vi "Configuration Utility.vi"() -> ()   [LabVIEW 2013, in "configuration library.lvlib"]
doc: "This is the main VI for the configuration editor."
uses:
  configuration library.lvlib
  Controls/StateCluster.ctl
  <vilib>/NI/Tag Bus Data Framework/Configuration Editor/Classes/SystemConfigRepo/SystemConfigRepo.lvclass
  <vilib>/NI/Configuration Framework/Node/NodeRef.ctl
  <vilib>/NI/Configuration Framework/Node/NISE_CEF_Node.lvclass
  subVI/SplashScreen/splash screen.ctl
  subVI/SplashScreen/notifier data.ctl
  <vilib>/NI/Configuration Framework/Node/StandardEvents.ctl
  <vilib>/NI/Configuration Framework/Node/UserEventRef.ctl
  <vilib>/NI/Configuration Framework/Controls/EventCluster.ctl
  <vilib>/NI/Configuration Framework/Node/NodeChangeEvent.ctl
  <vilib>/NI/Configuration Framework/Node/CacheState.ctl
  <vilib>/NI/Configuration Framework/Node/RefreshUIEvent.ctl
  <vilib>/NI/Configuration Framework/Node/StopEvent.ctl
  <vilib>/NI/Configuration Framework/glyph manager/glyph manager.ctl
  <vilib>/picture/picture.llb/imagedata.ctl
  Controls/add message.ctl
  Controls/MoveMessage.ctl
  <vilib>/NI/Tag Bus Data Framework/Configuration Editor/Classes/Systems/Systems.lvclass
  <vilib>/NI/Configuration Framework/Repository/NISE_CEF_Repository.lvclass
  <vilib>/NI/AMC/Create Single Message.vi
  <vilib>/NI/AMC/Update Message Routing Info.vi
  <vilib>/NI/AMC/Read Termination Message.vi
  <vilib>/NI/Tag Bus Data Framework/Configuration Editor/subVIs/Glyphs Status.ctl
  <vilib>/NI/Tag Bus Data Framework/Configuration Editor/subVIs/Add status to name.vi
  <vilib>/NI/AMC/Send Message.vi
  <vilib>/NI/AMC/Globals.vi
  <vilib>/NI/Tag Bus Data Framework/Configuration Editor/Classes/Module editor node/module editor node.lvclass
  <vilib>/NI/Tag Bus Data Framework/Configuration Editor/Classes/EngineTags/EngineTags.lvclass
  <vilib>/NI/Module Timing Source/timing source/TBM timing source.lvclass
  <vilib>/NI/Tag Bus Data Framework/Configuration Editor/Classes/TBM Configuration Node/TBM Configuration Node.lvclass
  <vilib>/NI/Tag Bus Module Framework/root configuration/TBM configuration.lvclass
  <vilib>/NI/Tag Bus Data Framework/Framework Configuration Classes/target configuration/PL_Target Configuration.lvclass
  <vilib>/NI/Tag Bus Data Framework/Configuration Editor/Classes/Targets/Targets.lvclass
  <vilib>/NI/Tag Bus Data Framework/Configuration Editor/Classes/Engine Parent/Engine Parent Editor Node.lvclass
  <vilib>/NI/Tag Bus Data Framework/Framework Configuration Classes/system configuration/PL_System Configuration.lvclass
  <vilib>/NI/Module Execution Interface/Engine Configuration/engine configuration.lvclass
  <vilib>/NI/Tag Bus Module Framework/channel/TBM channel.lvclass
  <vilib>/NI/Tag Bus Module Framework/module configuration/TBM module configuration.lvclass
  <vilib>/NI/AMC/AMC.lvlib
  <vilib>/NI/Configuration Framework/NISE_CEF_TreeControl.lvlib
  subVI/SplashScreen/splash screen.lvlib
  <vilib>/NI/Tag Bus Data Framework/Framework Configuration Classes/class cache/PL_class cache.lvlib
  <vilib>/NI/Tag Bus Data Framework/Configuration Editor/PL Framework Configuration Tool.lvlib
  <vilib>/NI/Configuration Framework/hierarchy repo/NISE_CEF_HierarchyRepo.lvclass
  <vilib>/NI/Configuration Framework/tree serializer/NISE_CEF_TreeSerializer.lvlib
  <vilib>/NI/Configuration Framework/glyph manager/glyph manager.lvlib
panel:
  in  "Exit":bool
  in  "View":string(tree)
  # "Tag Bus Configuration Editor"
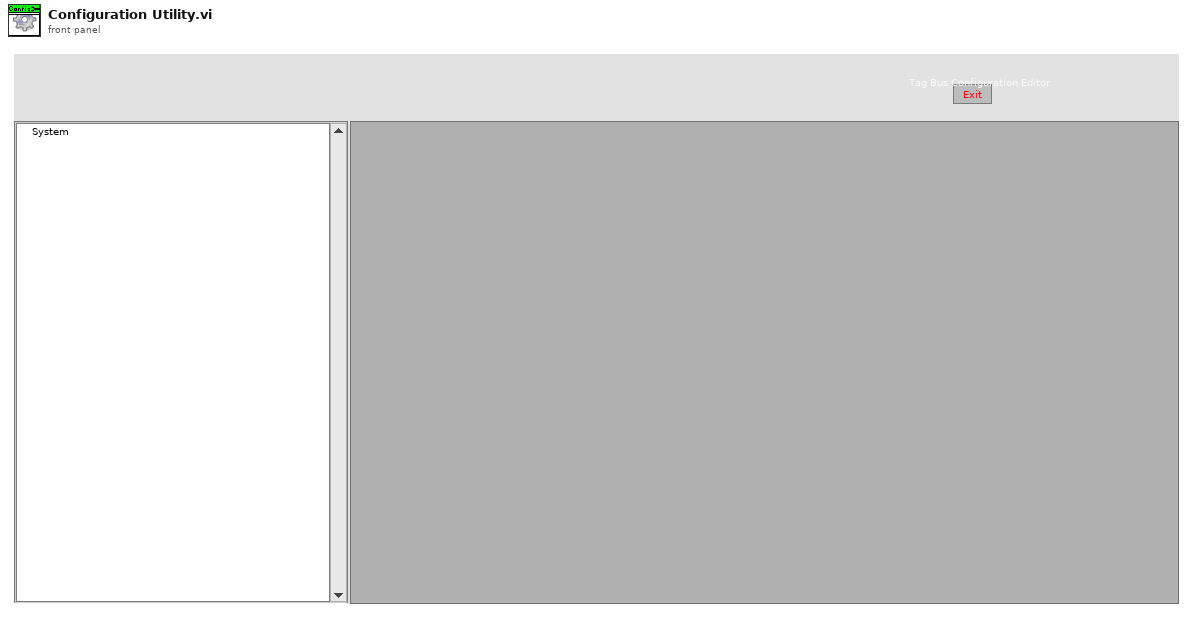
[diagram p1: front panel]
types:
  T1 = enum32{"Invalid", "Standard", "Closed", "Hidden", "Minimized", "Maximized"}
  T2 = typedef "configuration library.lvlib/StateCluster.ctl" = cluster{"repository":refnum<class "SystemConfigRepo.lvclass">, "root":T3, "unsaved changes":bool, "current path":path, "SplashScreen":T4, "classes cache":path, "standard events":T5, "glyph manager":T11}
  T3 = typedef "NISE_CEF_Node.lvclass/NodeRef.ctl" = refnum<data-value>
  T4 = typedef "configuration library.lvlib/splash screen.lvlib/splash screen.ctl" = cluster{"reference":refnum<vi>, "update notifier":refnum<notifier>, "Initialized":bool}
  T5 = typedef "NISE_CEF_Node.lvclass/StandardEvents.ctl" = cluster{"user event":T6, "node change":T7, "cache state":T8, "refresh UI":T9, "stop event":T10}
  T6 = typedef "NISE_CEF_Node.lvclass/UserEventRef.ctl" = refnum<user-event>
  T7 = typedef "NISE_CEF_Node.lvclass/NodeChangeEvent.ctl" = refnum<user-event>
  T8 = typedef "NISE_CEF_Node.lvclass/CacheState.ctl" = refnum<user-event>
  T9 = typedef "NISE_CEF_Node.lvclass/RefreshUIEvent.ctl" = refnum<user-event>
  T10 = typedef "NISE_CEF_Node.lvclass/StopEvent.ctl" = refnum<user-event>
  T11 = typedef "glyph manager.lvlib/glyph manager.ctl" = cluster{"search paths":path[], "glyph map":variant, "base glyphs":T12[], "desired overlays":string[]}
  T12 = typedef "imagedata.ctl" = cluster{"image type":i32, "image depth":i32, "image":u8[], "mask":u8[], "colors":u32[], "Rectangle":cluster{"left":i16, "top":i16, "right":i16, "bottom":i16}}
  T13 = typedef "AMC.lvlib/Message Queue.ctl" = refnum<queue>
  T14 = typedef "configuration library.lvlib/splash screen.lvlib/notifier data.ctl" = cluster{"Text":string, "percent":dbl}
  T15 = cluster{"node id":string, "RightClickPath":string}
  T16 = typedef "configuration library.lvlib/add message.ctl" = cluster{"node type":string, "to add to":string}
  T17 = typedef "configuration library.lvlib/MoveMessage.ctl" = cluster{"node ref":T3, "new parent":T3}
  T18 = typedef "configuration library.lvlib/FilePaths.ctl" = cluster{"glyphs":path[], "classes":path, "classes cache":path}
  T19 = typedef "PL_class cache.lvlib/cache definition.ctl" = cluster{"configuration":T20, "class cache data":T21}
  T20 = typedef "PL_class cache.lvlib/cache search configuration.ctl" = cluster{"Search Paths":path[], "Folders to Exclude":string[], "full class list":path[]}
  T21 = typedef "PL_class cache.lvlib/cached class information.ctl" = cluster{"targets":T22[], "engines":T23[], "modules":T23[], "ignored class list":path[]}
  T22 = typedef "PL_class cache.lvlib/target class metadata.ctl" = cluster{"file name":string, "fully qualified name":string, "menu display name":string, "configuration class name":string}
  T23 = typedef "PL_class cache.lvlib/class metadata.ctl" = cluster{"file name":string, "fully qualified name":string, "menu display name":string, "configuration class":string, "instances allowed":i32, "supported targets":T24[]}
  T24 = typedef "TBM configuration.lvclass/Target Types.ctl" = enum16{"Windows", "Mac", "Linux", "Linux RT ARM", "VxWorks", "Pharlap", "Other", "Linux RT x64"}
  T25 = typedef "NISE_CEF_Node.lvclass/Summary.ctl" = cluster{"ID":string, "parent ID":string, "node type":string, "text":string, "additional text":string, "glyph":string, "depth":i32, "glyph overlay":string}
  T26 = typedef "LVPoint32TypeDef.ctl" = cluster{"Horizontal":i32, "Vertical":i32}
  T27 = cluster{"data name":string, "drag data":variant}[]
  T28 = typedef "NISE_CEF_Node.lvclass/NodeMenuOptions.ctl" = cluster{"removable":bool, "movable":bool, "duplicate":bool}
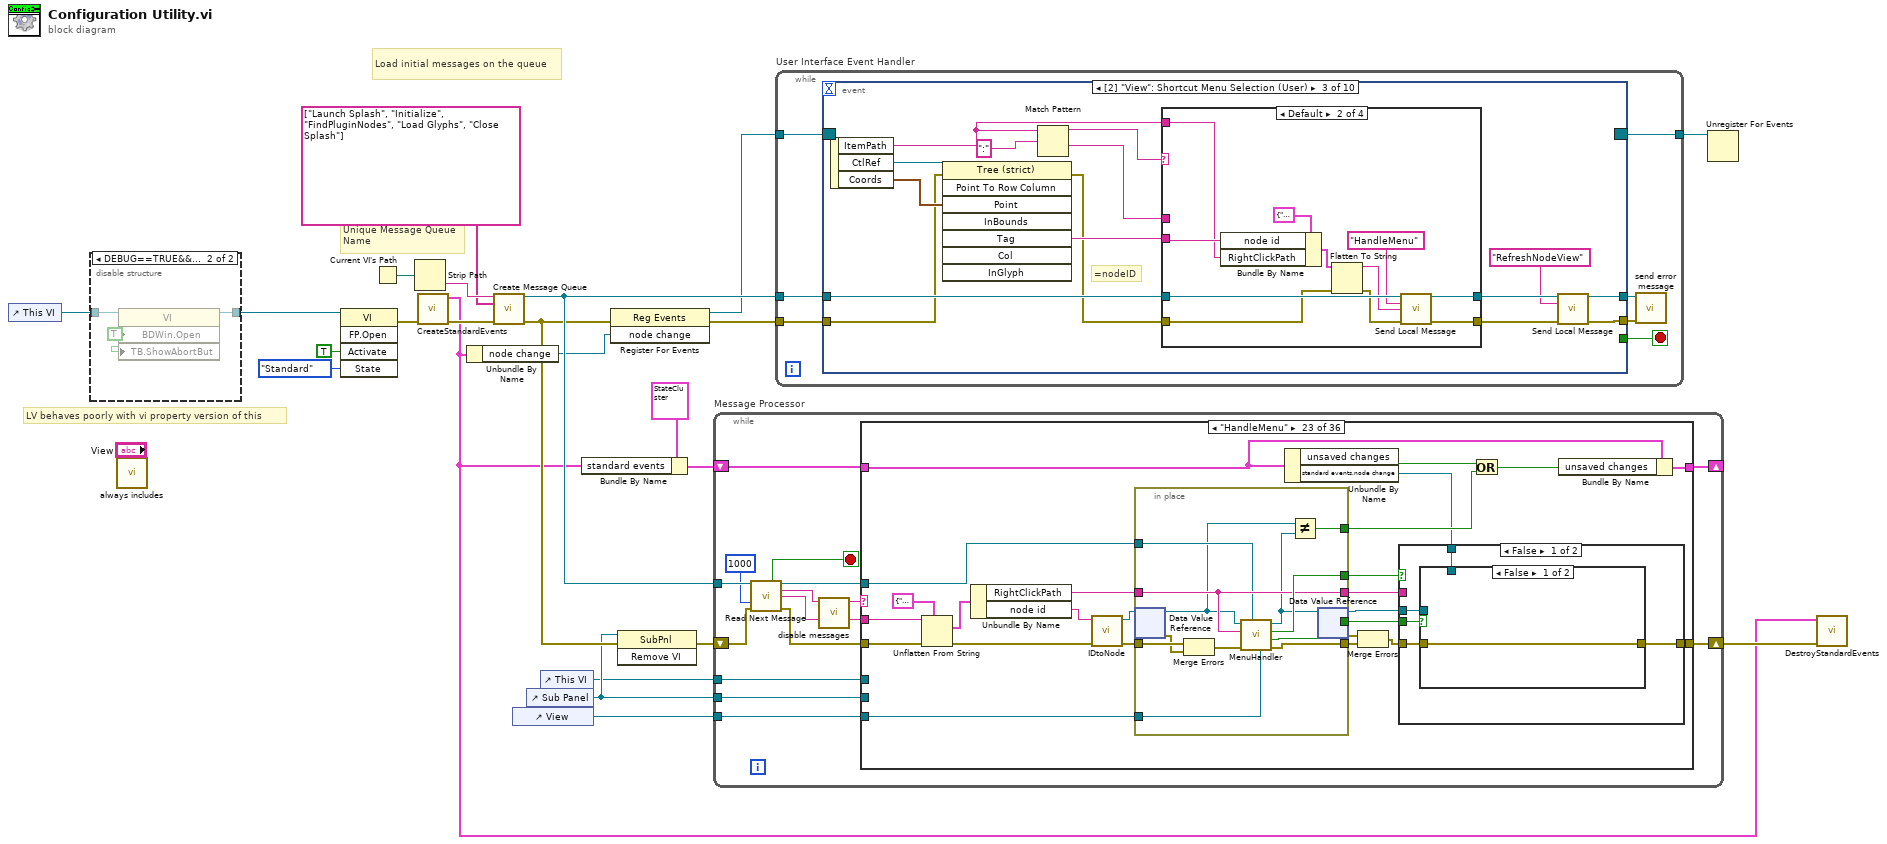
[diagram p0: block diagram]
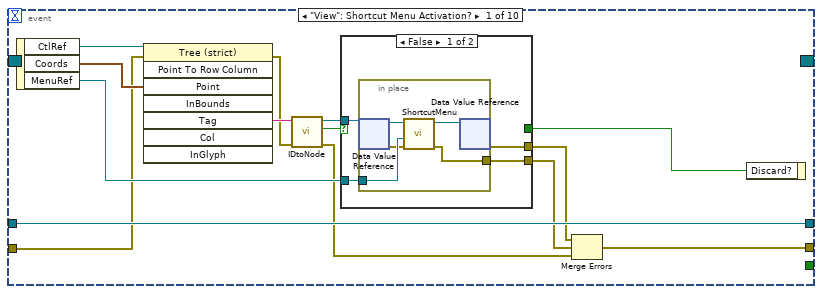
[diagram p3: hidden frame]
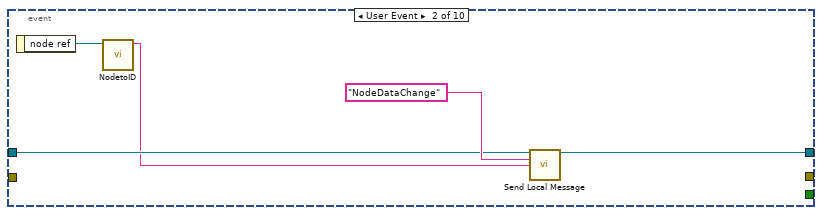
[diagram p5: hidden frame]
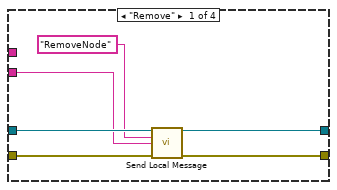
[diagram p6: hidden frame]
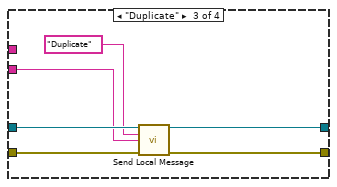
[diagram p7: hidden frame]
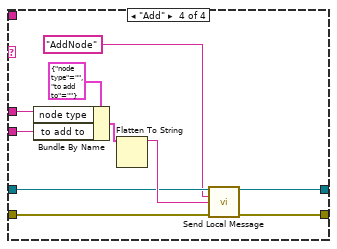
[diagram p8: hidden frame]
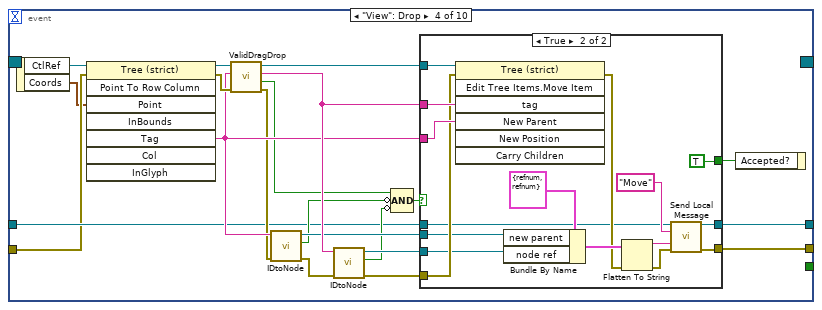
[diagram p9: hidden frame]
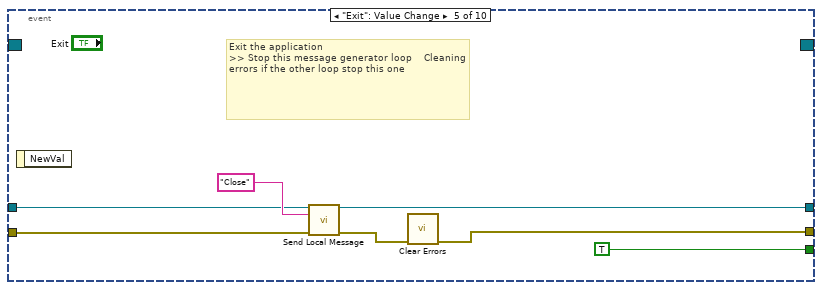
[diagram p11: hidden frame]
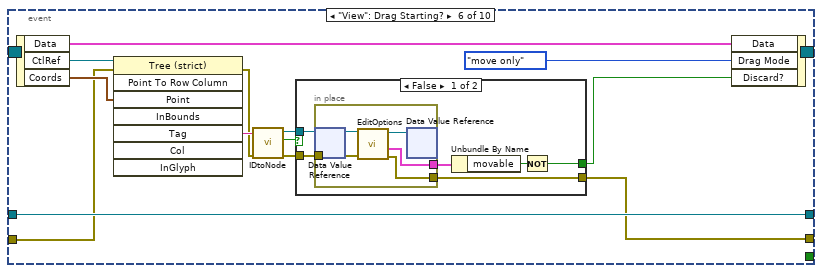
[diagram p12: hidden frame]
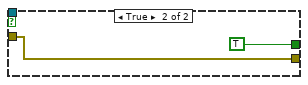
[diagram p13: hidden frame]
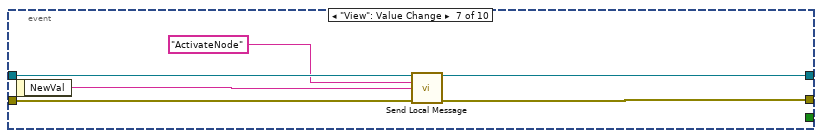
[diagram p14: hidden frame]
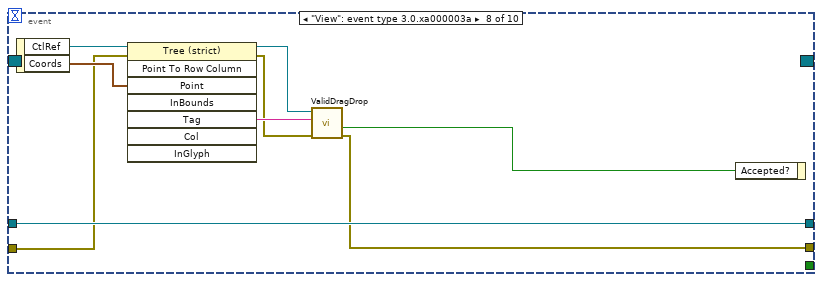
[diagram p15: hidden frame]
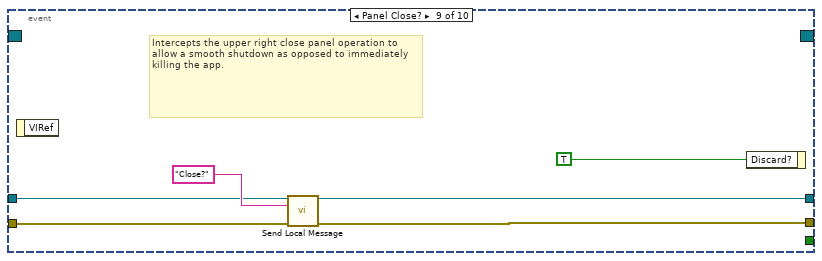
[diagram p16: hidden frame]
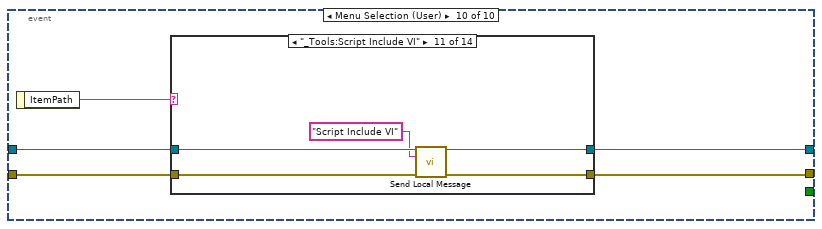
[diagram p17: hidden frame]
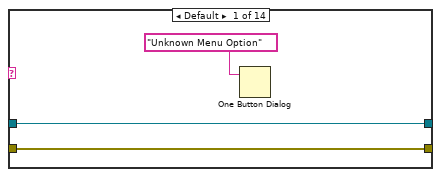
[diagram p18: hidden frame]
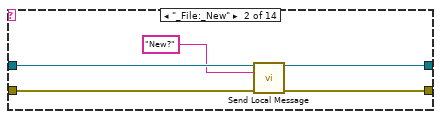
[diagram p19: hidden frame]
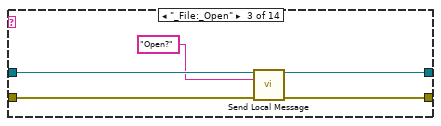
[diagram p20: hidden frame]
diagram:
  # "LV behaves poorly with vi property version of this"
  # "Unique Message Queue Name"
  # "Load initial messages on the queue"
  n1 = control-ref of="This VI"() -> (w14:refnum<vi>)
  n2 = disable-structure shown="DEBUG==TRUE&&RUN_TIME_ENGINE==False" {
    disable-tunnel: [w24 w27] -> w15
    disable-tunnel: w14 -> [w24 w26]
    frame condition #0 (active) {
    }
    frame condition #1 {
      w25 = TRUE ("Block Diagram Window:Open")
      n3 = property class="VI"(reference=w26, "BDWin.Open"=w25, "TB.ShowAbortBut"=w25) -> (reference out=w27:refnum<vi>)  [unwired: 1 in, 1 out]
    }
  }
  n4 = call "always includes.vi"() -> ()  [unwired: 12 in]
  n5 = invoke class="VI" method="FP.Open"(reference=w15, "Activate"=TRUE ("Activate?"), "State"=T1."Standard") -> (error out=w9:errorcluster)  [unwired: 2 in, 4 out]
  n6 = Current VI's Path() -> (path=w22:path)
  n7 = Strip Path(path=w22) -> (name=w23:string)  [unwired: 1 out]
  n8 = call <vilib>:"CreateStandardEvents.vi"("error in"=w9) -> ("error out"=w8:errorcluster, "standard events"=w1:T5)  [unwired: 9 in]
  n9 = Unbundle By Name(w1) -> ("node change"=w6:T7)
  n10 = call <vilib>:"Create Message Queue.vi"("message queue name"=w23, "initial message names"=string[] ["Launch Splash", "Initialize", "FindPluginNodes", "Load Glyphs", "Close Splash"], "error in"=w8) -> ("message queue out"=w20:T13, "error out"=w18:errorcluster)  [unwired: 11 in]
  n11 = control-ref of="View"() -> (w13:refnum<vi>)
  n12 = control-ref of="Sub Panel"() -> (w11:refnum<vi>)
  n13 = control-ref of="This VI"() -> (w10:refnum<vi>)
  n14 = Bundle By Name(cluster=T2 {"repository"=refnum, "root"=refnum, "unsaved changes"=FALSE, "current path"=path "", "SplashScreen"={"reference"=refnum, "update notifier"=refnum, "Initialized"=FALSE}, "classes cache"=path "", "standard events"={"user event"=refnum, "node change"=refnum, "cache state"=refnum, "refresh UI"=refnum, "stop event"=refnum}, "glyph manager"={"search paths"=[], "glyph map"=variant, "base glyphs"=[], "desired overlays"=[]}}, "standard events"=w1) -> (w4:T2)
  n15 = register-events(error in=w18, w6) -> (reference out=w5:refnum<event-registration>, error out=w7:errorcluster)  [unwired: 1 in]
  n16 = invoke class="SubPnl" method="Remove VI"(reference=w11, error in=w18) -> (error out=w12:errorcluster)  [unwired: 1 in, 2 out]
  n17 = while "Message Processor" {
    shift-right: [w40] -> w2
    shift-left: w12 -> [w39]
    tunnel: w20 -> [w38]
    shift-right: [w36] -> _
    shift-left: w4 -> [w35]
    tunnel: w10 -> [w30]
    tunnel: w11 -> [w29]
    tunnel: w13 -> [w28]
    stop <- w42 stop-if-true
    n18 = call <vilib>:"Read Next Message.vi"("message queue in"=w38, "timeout (1 ms)"=1000, "error in"=w39) -> ("exit process?"=w42:bool, "message queue out"=w34:T13, "message name"=w31:string, "message value"=w33:string, "error out"=w41:errorcluster)  [unwired: 5 in, 3 out]
    n19 = call "disable messages.vi"("message to check"=w31) -> ("message out"=w32:string)  [unwired: 10 in]
    n20 = case shown="\"HandleMenu\"" w32 {
      selector: w32 -> [_ w46 _ _ _ _ _ _ _ _ _ w165 _ _ _ w288 _ _ _ _ _ _ _ _ _ _ _ _ _ _ _ _ _ _ _ _]
      tunnel: w33 -> [_ _ _ _ _ _ _ _ w121 _ _ _ _ _ _ _ _ w331 _ _ w400 _ w451 _ _ w512 w530 w553 _ w583 _ _ w638 w663 _ w672]
      tunnel: w41 -> [w44 w49 w51 w58 w71 w79 w106 w112 w122 w148 w152 w162 w189 w215 w250 w281 w308 w336 w353 w360 w398 w415 w452 w481 w484 w511 w529 w554 w569 w582 w616 w626 w637 w662 w669 w675]
      tunnel: [w44 w49 w51 w61 w68 w78 w107 w115 errorcluster {"status"=FALSE, "code"=0, "source"=""} ("error out") w146 w152 w167 w206 w208 w243 w291 w318 w335 w352 w362 w385 w414 w440 w480 w484 w493 w531 w556 w569 w581 w613 w624 w636 w661 w667 w674] -> w40
      tunnel: [w43 w45 w50 w59 w63 w77 w97 w113 w123 w145 w151 w163 w204 w207 w242 w292 w319 w332 w354 w361 w401 w411 w437 w482 w483 w496 w524 w555 w570 w573 w605 w625 w634 w652 w668 w671] -> w36
      tunnel: w35 -> [w43 w45 w50 w60 w72 w87 w98 w113 w123 w145 w151 w164 w188 w216 w251 w287 w314 w333 w354 w361 w401 w412 w438 w482 w483 w510 w522 w548 w571 w575 w621 w625 w634 w664 w668 w677]
      tunnel: w34 -> [_ _ _ _ _ _ w108 w114 w125 w147 _ w166 w205 w214 w249 w278 w317 w334 _ w363 _ w413 w442 _ _ _ _ _ _ _ _ _ w635 w660 _ w673]
      tunnel: w30 -> [_ _ _ w52 w67 _ w95 _ _ _ _ _ _ _ _ _ _ _ _ _ _ _ _ _ _ _ _ _ _ _ w612 _ _ _ _ _]
      tunnel: w29 -> [_ _ _ _ _ _ _ _ w117 w139 _ w154 _ _ _ w279 w306 _ _ _ _ _ _ _ _ _ _ _ _ w576 _ w623 w627 _ _ _]
      tunnel: w28 -> [_ _ _ _ _ w75 _ _ _ _ _ w153 _ _ _ _ _ _ _ _ _ _ w441 _ _ w497 w525 w549 _ w577 w615 _ _ _ _ _]
      frame "", "Idle" {
      }
      frame "Missing Message Handler", Default {
        # "Call this case if a message is received that is not handled by any other case. Typically this is a programming error as a result of a typo or unhandled message/missing message handler."
        n21 = Format Into String(format string="Internal Error: Missing message handler for '%s\" message." ("message"), w46) -> (resulting string=w48:string)  [unwired: 2 in, 1 out]
        n22 = One Button Dialog(message=w48) -> ()  [unwired: 2 out]
      }
      frame "------------Generic Operations------------" {
        # "Dummy case to add a seperation in the Case Structure menu"
      }
      frame "Launch Splash" {
        n23 = invoke class="VI" method="FP.Center"(reference=w52, error in=w58) -> (reference out=w56:refnum<vi>, error out=w55:errorcluster)  [unwired: 1 in, 1 out]
        n24 = invoke class="VI" method="FP.Open"(reference=w56, error in=w55, "State"=T1."Hidden") -> (error out=w53:errorcluster)  [unwired: 2 in, 4 out]
        n25 = call "Launch.vi"("error in"=w53) -> ("error out"=w61:errorcluster, "SplashScreen"=w57:T4)  [unwired: 9 in]
        n26 = Bundle By Name(cluster=w60, "SplashScreen"=w57) -> (w59:T2)
      }
      frame "Initialize" {
        # "issues in exe"
        n27 = Current VI's Menubar() -> (w70:refnum<k9>)
        n28 = call "menu options.vi"("error in"=w71, "VI ref"=w67, "menu ref in"=w70) -> ("error out"=w68:errorcluster)  [unwired: 7 in, 1 out]
        n29 = call "default file paths.vi"() -> ("paths"=w69:T18)  [unwired: 11 in]
        n30 = Unbundle By Name(w69) -> ("classes cache"=w66:path)
        n31 = Bundle By Name(cluster=w72, "classes cache"=w66) -> (w63:T2)
        n32 = Unbundle By Name(w63) -> ("SplashScreen"=w62:T4)
        n33 = call "Update.vi"("Update"=T14 {"Text"="Preparing UI...", "percent"=27.0}, "SplashScreen in"=w62) -> ("error out"=w65:errorcluster)  [unwired: 8 in, 1 out]
        n34 = call <vilib>:"Clear Errors.vi"("error in (no error)"=w65) -> ()  [unwired: 6 in, 1 out]
      }
      frame "Load Glyphs" {
        n35 = Unbundle By Name(w87) -> ("SplashScreen"=w86:T4)
        n36 = call "default file paths.vi"() -> ("paths"=w74:T18)  [unwired: 11 in]
        n37 = invoke class="Tree (strict)" method="Custom Item Symbols.Revert Symbols"(reference=w75, error in=w79) -> (reference out=w85:refnum<vi>, error out=w84:errorcluster)  [unwired: 1 in, 1 out]
        n38 = Unbundle By Name(w74) -> ("glyphs"=w73:path[])
        n39 = call <vilib>:"create glyph manager.vi"("error in"=w84, "tree ref (for default symbols)"=w85) -> ("error out"=w80:errorcluster, "glyph manager"=w81:T11)  [unwired: 8 in]
        n40 = call "Update.vi"("Update"=T14 {"Text"="Loading Glyphs...", "percent"=78.0}, "SplashScreen in"=w86) -> ("error out"=w89:errorcluster)  [unwired: 8 in, 1 out]
        n41 = for {
          tunnel: w73 -> [w90] mode=indexing
          shift-right: [w94] -> w83
          shift-left: w81 -> [w92]
          shift-right: [w93] -> w82
          shift-left: w80 -> [w91]
          n42 = call <vilib>:"add search path.vi"("error in"=w91, "search path"=w90, "glyph manager in"=w92) -> ("error out"=w93:errorcluster, "glyph manager out"=w94:T11)  [unwired: 7 in]
        }
        n43 = call <vilib>:"Clear Errors.vi"("error in (no error)"=w89) -> ()  [unwired: 6 in, 1 out]
        n44 = call <vilib>:"update tree control.vi"("error in"=w82, "tree reference"=w85, "glyph manager in"=w83) -> ("error out"=w78:errorcluster, "glyph manager out"=w76:T11)  [unwired: 7 in]
        n45 = Bundle By Name(cluster=w87, "glyph manager"=w76) -> (w77:T2)
      }
      frame "Close Splash" {
        n46 = Unbundle By Name(w98) -> ("SplashScreen"=w104:T4)
        n47 = call "Close.vi"("error in"=w106, "SplashScreen"=w104) -> ("error out"=w100:errorcluster, "SplashScreen out"=w96:T4)  [unwired: 8 in]
        n48 = Bundle By Name(cluster=w98, "SplashScreen"=w96) -> (w97:T2)
        n49 = invoke class="VI" method="FP.Open"(reference=w95, error in=w100, "State"=T1."Standard") -> (reference out=w102:refnum<vi>, error out=w101:errorcluster)  [unwired: 2 in, 3 out]
        n50 = Close Reference(reference=w102, error in (no error)=w101) -> (error out=w99:errorcluster)
        n51 = call <vilib>:"Send Local Message.vi"("message queue in"=w108, "message name"="New" ("Message Name"), "error in"=w99) -> ("error out"=w107:errorcluster)  [unwired: 10 in, 2 out]
      }
      frame "Close" {
        n52 = Unbundle By Name(w113) -> ("root"=w110:T3)
        n53 = call <vilib>:"CloseNode.vi"("error in"=w112, "node ref"=w110) -> ("error out"=w109:errorcluster)  [unwired: 9 in]
        n54 = call <vilib>:"Send Local Message.vi"("message queue in"=w114, "message name"="Exit", "error in"=w109) -> ("error out"=w115:errorcluster)  [unwired: 10 in, 2 out]
      }
      frame "Error" {
        n55 = Unbundle By Name(w123) -> ("standard events"=w116:T5)
        n56 = call "Remove UI without races.vi"("error in"=w122, "standard events"=w116, "sub panel ref in"=w117) -> ("error out"=w118:errorcluster)  [unwired: 7 in, 1 out]
        n57 = case shown="\"\"" w121 {
          selector: w121 -> [w127 _]
          tunnel: w122 -> [w128 w129]
          tunnel: [w126 w129] -> w119
          frame Default {
            n58 = Unflatten From String(type=w128, binary string=w127, error in (no error)=w128) -> (value=w126:errorcluster)  [unwired: 2 in, 2 out]
          }
          frame "" {
          }
        }
        n59 = call <vilib>:"Clear Errors.vi"("error in (no error)"=w118) -> ()  [unwired: 6 in, 1 out]
        n60 = Unbundle By Name(w119) -> ("code"=w120:i32)
        n61 = case shown="15550" w120 {
          tunnel: w125 -> [_ _ _ w135 _]
          tunnel: w119 -> [_ _ _ w134 w137]
          frame -2147220623, -2147220621, -2147220364, 56, 63 {
            n62 = One Button Dialog(message="Problem communicating with remote device.  Make sure a valid device is selected and that the IP address is correct.") -> ()  [unwired: 1 in, 1 out]
          }
          frame 1003 {
            n63 = One Button Dialog(message="Dev Error: The Ui.vi for the selected class is broken") -> ()  [unwired: 1 in, 1 out]
          }
          frame 15550 {
            n64 = One Button Dialog(message="The cRIO does not yet have a configuration to download. Create or open a configuration and download it to the cRIO") -> ()  [unwired: 1 in, 1 out]
          }
          frame 537549 {
            n65 = call <vilib>:"Send Local Message.vi"("message queue in"=w135, "message name"="Exit", "error in"=w134) -> ()  [unwired: 10 in, 3 out]
            n66 = One Button Dialog(message="Invalid configuration file.") -> ()  [unwired: 1 in, 1 out]
          }
          frame 1, Default {
            n67 = call <vilib>:"Simple Error Handler.vi"("error in (no error)"=w137) -> ()  [unwired: 1 in, 8 out]
          }
        }
      }
      frame "Exit" {
        # "Stop the VI                                                                             >> Perform any cleanup tasks in this message case. >> Clear display before closing."
        n68 = call <vilib>:"Destroy Message Queue.vi"("message queue in"=w147, "error in"=w148) -> ("error out"=w142:errorcluster)  [unwired: 11 in, 2 out]
        n69 = control-ref of="Exit"() -> (w144:refnum<vi>)
        n70 = Unbundle By Name(w145) -> ("standard events"=w138:T5)
        n71 = property class="Bool (strict)"(reference=w144, error in=w142, "Val(Sgnl)"=FALSE ("Exit")) -> (error out=w141:errorcluster)  [unwired: 1 out]
        n72 = call "Remove UI without races.vi"("error in"=w141, "standard events"=w138, "sub panel ref in"=w139) -> ("error out"=w140:errorcluster)  [unwired: 7 in, 1 out]
        n73 = disable-structure shown="RUN_TIME_ENGINE==True" {
          disable-tunnel: [w149 w150] -> w146
          disable-tunnel: w140 -> [w149 w150]
          frame condition #0 (active) {
          }
          frame condition #1 {
            n74 = Quit LabVIEW() -> ()  [unwired: 1 in]
          }
        }
      }
      frame "------------Menu Operations--------------" {
        # "Dummy case to add a seperation in the Case Structure menu"
      }
      frame "Close?", "New?", "Open?" {
        n75 = Unbundle By Name(w164) -> ("unsaved changes"=w155:bool, "standard events"=w156:T5)
        n76 = case shown="True" w155 {
          tunnel: [TRUE ("SaveFlag") w185] -> w158
          tunnel: w164 -> [w177 w184]
          tunnel: [w177 w183] -> w163
          tunnel: w162 -> [w176 w182]
          tunnel: [w176 w181] -> w157
          tunnel: w154 -> [_ w180]
          tunnel: w153 -> [_ w179]
          frame False {
            # "If there is nothing to save Go do Action"
          }
          frame True {
            n77 = call "dialog save dirty dot.vi"("error in"=w182, "View"=w179, "sub panel ref in"=w180, "state in"=w184) -> ("error out"=w181:errorcluster, "new"=w185:bool, "state out"=w183:T2)  [unwired: 5 in]
          }
        }
        n78 = Search and Replace String(input string=w165, search string="?", replace string="") -> (result string=w159:string)  [unwired: 5 in, 3 out]
        n79 = case shown="True" w158 {
          tunnel: w157 -> [w168 w175]
          tunnel: [w168 w171] -> w167
          tunnel: w166 -> [_ w174]
          tunnel: w159 -> [_ w173]
          tunnel: w156 -> [_ w169]
          tunnel: w154 -> [_ w170]
          frame False {
          }
          frame True {
            n80 = call <vilib>:"Send Local Message.vi"("message queue in"=w174, "message name"=w173, "error in"=w175) -> ("error out"=w172:errorcluster)  [unwired: 10 in, 2 out]
            n81 = call "Remove UI without races.vi"("error in"=w172, "standard events"=w169, "sub panel ref in"=w170) -> ("error out"=w171:errorcluster)  [unwired: 7 in, 1 out]
          }
        }
      }
      frame "New" {
        # "unused"
        n82 = Unbundle By Name(w188) -> ("glyph manager"=w187:T11)
        n83 = call <vilib>:"create default cache.vi"() -> ("cache"=w195:T19)  [unwired: 11 in]
        n84 = Unbundle By Name(w195) -> ("configuration.Search Paths"=w194:path[])
        n85 = call-dynamic "AddGlyphtoGManager.vi"("error in"=w189, "glyph manager"=w187, "NISE_CEF_serializable node in"=refnum<class "Systems.lvclass"> refnum ("Systems.lvclass")) -> ("error out"=w190:errorcluster, "glyph manager out"=w186:T11, "NISE_CEF_serializable node out"=w191:refnum<class "Systems.lvclass">)  [unwired: 6 in]
        n86 = call-dynamic "Initialize.vi"("error in"=w190, "node in"=w191) -> ("error out"=w200:errorcluster, "data value reference"=w201:T3)  [unwired: 7 in, 1 out]
        n87 = Delete From Array(array=w194) -> (deleted portion=w193:path)  [unwired: 2 in, 1 out]
        n88 = call-dynamic "Initialize.vi"("error in"=w200, "path"=w193, "repository in"=refnum<class "SystemConfigRepo.lvclass"> refnum ("SystemConfigRepo.lvclass")) -> ("error out"=w199:errorcluster, "repository out"=w198:refnum<class "SystemConfigRepo.lvclass">)  [unwired: 7 in]
        n89 = Bundle By Name(cluster=w188, "unsaved changes"=FALSE ("SaveFlag"), "repository"=w198, "root"=w201, "current path"=path "", "glyph manager"=w186) -> (w204:T2)
        n90 = call <vilib>:"Send Local Message.vi"("message queue in"=w205, "message name"="PopulateTree", "error in"=w199) -> ("error out"=w206:errorcluster)  [unwired: 10 in, 2 out]
      }
      frame "Open" {
        n91 = call <vilib>:"Set Busy.vi"() -> ("error out"=w211:errorcluster)  [unwired: 10 in, 1 out]
        n92 = call "File Dialog"("pattern (all files)"="*.pcfg") -> ("selected path"=w213:path, "cancelled"=w212:bool)  [unwired: 11 in, 2 out]
        n93 = case shown="False" w212 {
          tunnel: w216 -> [w225 w241]
          tunnel: [w224 w241] -> w207
          tunnel: w215 -> [w223 w240]
          tunnel: w214 -> [w222 _]
          tunnel: [w221 w240] -> w208
          tunnel: w213 -> [w218 _]
          tunnel: w211 -> [w217 w239]
          tunnel: [w217 w239] -> w210
          frame False {
            n94 = in-place {
              in-place-border: w223 -> [w238]
              in-place-border: [w227] -> w219
              in-place-border: w218 -> [w233]
              n95 = in-place-cluster #1(w225) -> ("repository"=w226:refnum<class "SystemConfigRepo.lvclass">, "current path"=w234:path)  [unwired: 2 out]
              n96 = call-dynamic "Open.vi"("error in"=w238, "file path"=w233, "repository in"=w226) -> ("error out"=w235:errorcluster, "repository out"=w231:refnum<class "SystemConfigRepo.lvclass">)  [unwired: 6 in, 1 out]
              n97 = call-dynamic "WriteTree.vi"("error in"=w235, "repository in"=w231) -> ("error out"=w228:errorcluster, "root"=w236:T3, "repository out"=w230:refnum<class "NISE_CEF_Repository.lvclass">)  [unwired: 7 in]
              n98 = To More Specific Class(target class=w226, reference=w230, error in=w228) -> (specific class reference=w229:refnum<class "SystemConfigRepo.lvclass">, error out=w227:errorcluster)
              n99 = Select(t=w234, s=w227, f=w233) -> (s? t:f=w232:path)
              n100 = in-place-cluster #1("unsaved changes"=FALSE ("SaveFlag"), "repository"=w229, "root"=w236, "current path"=w232) -> (w224:T2)
            }
            n101 = call <vilib>:"Send Local Message.vi"("message queue in"=w222, "message name"="PopulateTree", "error in"=w219) -> ("error out"=w221:errorcluster)  [unwired: 10 in, 2 out]
          }
          frame True {
          }
        }
        n102 = call <vilib>:"Unset Busy.vi"("error in (no error)"=w210) -> ()  [unwired: 10 in, 1 out]
      }
      frame "Load Binary" {
        n103 = call <vilib>:"Set Busy.vi"() -> ("error out"=w246:errorcluster)  [unwired: 10 in, 1 out]
        n104 = call "File Dialog2"("pattern (all files)"="*.pbin") -> ("selected path"=w248:path, "cancelled"=w247:bool)  [unwired: 11 in, 2 out]
        n105 = case shown="False" w247 {
          tunnel: w251 -> [w260 w276]
          tunnel: [w259 w276] -> w242
          tunnel: w250 -> [w258 w275]
          tunnel: w249 -> [w257 _]
          tunnel: [w256 w275] -> w243
          tunnel: w248 -> [w253 _]
          tunnel: w246 -> [w252 w274]
          tunnel: [w252 w274] -> w245
          frame False {
            n106 = in-place {
              in-place-border: w258 -> [w263]
              in-place-border: [w268] -> w254
              in-place-border: w253 -> [w264]
              n107 = in-place-cluster #2(w260) -> ("repository"=w265:refnum<class "SystemConfigRepo.lvclass">)  [unwired: 2 out]
              n108 = call <vilib>:"read full file.vi"("error in"=w263, "file path"=w264) -> ("error out"=w262:errorcluster, "data"=w261:string)  [unwired: 8 in]
              n109 = call <vilib>:"unflatten memory.vi"("error in"=w262, "binary repo"=w261, "NISE_CEF_HierarchyRepo in"=w265) -> ("error out"=w266:errorcluster, "NISE_CEF_HierarchyRepo out"=w267:refnum<class "SystemConfigRepo.lvclass">)  [unwired: 7 in]
              n110 = call-dynamic "WriteTree.vi"("error in"=w266, "repository in"=w267) -> ("error out"=w269:errorcluster, "root"=w272:T3, "repository out"=w271:refnum<class "NISE_CEF_Repository.lvclass">)  [unwired: 7 in]
              n111 = To More Specific Class(target class=w265, reference=w271, error in=w269) -> (specific class reference=w270:refnum<class "SystemConfigRepo.lvclass">, error out=w268:errorcluster)
              n112 = in-place-cluster #2("unsaved changes"=TRUE ("SaveFlag"), "repository"=w270, "root"=w272) -> (w259:T2)
            }
            n113 = call <vilib>:"Send Local Message.vi"("message queue in"=w257, "message name"="PopulateTree", "error in"=w254) -> ("error out"=w256:errorcluster)  [unwired: 10 in, 2 out]
          }
          frame True {
          }
        }
        n114 = call <vilib>:"Unset Busy.vi"("error in (no error)"=w245) -> ()  [unwired: 10 in, 1 out]
      }
      frame "Save", "SaveAs" {
        n115 = Unbundle By Name(w287) -> ("standard events"=w277:T5)
        n116 = call <vilib>:"Set Busy.vi"() -> ("error out"=w285:errorcluster)  [unwired: 10 in, 1 out]
        n117 = call "Remove UI without races.vi"("error in"=w281, "standard events"=w277, "sub panel ref in"=w279) -> ("error out"=w280:errorcluster)  [unwired: 7 in, 1 out]
        n118 = flat-sequence {
          tunnel: w280 -> [w299]
          tunnel: w288 -> [w297]
          tunnel: w287 -> [w294]
          tunnel: w285 -> [w293]
          tunnel: [w300] -> w284
          tunnel: [w298] -> w283
          tunnel: [w293] -> w282
          tunnel: [w302] -> w286
          tunnel: [w303] -> w289
          tunnel: [w304] -> w292
          tunnel: w284 -> [w304]
          tunnel: w283 -> [w303]
          tunnel: w282 -> [w302]
          frame #0 {
            n119 = Equal?(x="SaveAs", y=w297) -> (x = y?=w296:bool)
            n120 = call "save operation.vi"("force save as"=w296, "error in"=w299, "state cluster"=w294) -> ("error out"=w298:errorcluster, "state out"=w300:T2)  [unwired: 7 in]
          }
          frame #1 {
            n121 = local read "View"() -> (w301:string)
            n122 = property on="View" class="Tree (strict)"("Val(Sgnl)"=w301) -> ()  [unwired: 2 in, 2 out]
          }
        }
        n123 = call <vilib>:"Unset Busy.vi"("error in (no error)"=w286) -> ()  [unwired: 10 in, 1 out]
        n124 = call <vilib>:"Send Local Message.vi"("message queue in"=w278, "message name"="PopulateTree", "error in"=w289) -> ("error out"=w291:errorcluster)  [unwired: 10 in, 2 out]
      }
      frame "Save Binary" {
        n125 = Unbundle By Name(w314) -> ("standard events"=w305:T5)
        n126 = call <vilib>:"Set Busy.vi"() -> ("error out"=w312:errorcluster)  [unwired: 10 in, 1 out]
        n127 = call "Remove UI without races.vi"("error in"=w308, "standard events"=w305, "sub panel ref in"=w306) -> ("error out"=w307:errorcluster)  [unwired: 7 in, 1 out]
        n128 = flat-sequence {
          tunnel: w307 -> [w323]
          tunnel: w314 -> [w320]
          tunnel: w312 -> [w324]
          tunnel: [w321] -> w311
          tunnel: [w322] -> w310
          tunnel: [w324] -> w309
          tunnel: [w326] -> w313
          tunnel: [w327] -> w315
          tunnel: [w328] -> w319
          tunnel: w311 -> [w328]
          tunnel: w310 -> [w327]
          tunnel: w309 -> [w326]
          frame #0 {
            n129 = call "save operation binary.vi"("error in"=w323, "state cluster"=w320) -> ("error out"=w322:errorcluster, "state out"=w321:T2)  [unwired: 8 in]
          }
          frame #1 {
            n130 = local read "View"() -> (w325:string)
            n131 = property on="View" class="Tree (strict)"("Val(Sgnl)"=w325) -> ()  [unwired: 2 in, 2 out]
          }
        }
        n132 = call <vilib>:"Unset Busy.vi"("error in (no error)"=w313) -> ()  [unwired: 10 in, 1 out]
        n133 = call <vilib>:"Send Local Message.vi"("message queue in"=w317, "message name"="PopulateTree", "error in"=w315) -> ("error out"=w318:errorcluster)  [unwired: 10 in, 2 out]
      }
      frame "Custom View" {
        n134 = in-place {
          in-place-border: w336 -> [w349]
          in-place-border: [w340] -> w329
          in-place-border: w331 -> [w341]
          n135 = in-place-cluster #3(w333) -> ("repository"=w338:refnum<class "SystemConfigRepo.lvclass">, "root"=w347:T3)
          n136 = call-dynamic "ReadTree.vi"("error in"=w349, "root"=w347, "repository in"=w338) -> ("error out"=w345:errorcluster, "repository out"=w343:refnum<class "NISE_CEF_Repository.lvclass">)  [unwired: 7 in]
          n137 = call-dynamic "CustomView.vi"("error in"=w345, "view name"=w341, "repository in"=w343) -> ("error out"=w344:errorcluster, "repository out"=w342:refnum<class "NISE_CEF_Repository.lvclass">)  [unwired: 7 in]
          n138 = call-dynamic "WriteTree.vi"("error in"=w344, "repository in"=w342) -> ("error out"=w348:errorcluster, "root"=w346:T3, "repository out"=w339:refnum<class "NISE_CEF_Repository.lvclass">)  [unwired: 7 in]
          n139 = To More Specific Class(target class=w338, reference=w339, error in=w348) -> (specific class reference=w337:refnum<class "SystemConfigRepo.lvclass">, error out=w340:errorcluster)
          n140 = in-place-cluster #3("repository"=w337, "root"=w346) -> (w332:T2)
        }
        n141 = call <vilib>:"Send Local Message.vi"("message queue in"=w334, "message name"="PopulateTree", "error in"=w329) -> ("error out"=w335:errorcluster)  [unwired: 10 in, 2 out]
      }
      frame "DeployTool" {
        n142 = Unbundle By Name(w354) -> ("current path"=w350:path, "root"=w351:T3)
        n143 = call <vilib>:"deployment tool.vi"("current pcfg path"=w350, "error in"=w353, "root"=w351) -> ("error out"=w352:errorcluster)  [unwired: 8 in]
      }
      frame "Edit Plugin Search Paths" {
        n144 = Unbundle By Name(w361) -> ("classes cache"=w359:path)
        n145 = call <vilib>:"load cache.vi"("error in"=w360, "cache path"=w359) -> ("error out"=w358:errorcluster, "cache"=w356:T19)  [unwired: 8 in]
        n146 = case shown="No Error" w358 {
          selector: w358 -> [w368 w371]
          tunnel: [w369 w372] -> w357
          tunnel: w356 -> [w369 _]
          tunnel: [w368 w370] -> w355
          frame No Error {
          }
          frame Error {
            n147 = call <vilib>:"create default cache.vi"() -> ("cache"=w372:T19)  [unwired: 11 in]
            n148 = call <vilib>:"Clear Errors.vi"("error in (no error)"=w371) -> ("error out"=w370:errorcluster)  [unwired: 6 in]
          }
        }
        n149 = Unbundle By Name(w357) -> ("configuration.Search Paths"=w367:path[])
        n150 = call "dialog edit search paths.vi"("error in"=w355, "Plugin Search Paths"=w367) -> ("error out"=w364:errorcluster, "Cancelled?"=w366:bool, "Plugin Search Paths"=w365:path[])  [unwired: 7 in]
        n151 = case shown="False" w366 {
          tunnel: w357 -> [w382 _]
          tunnel: w365 -> [w381 _]
          tunnel: w364 -> [w375 w383]
          tunnel: w363 -> [w378 _]
          tunnel: [w377 w383] -> w362
          tunnel: w359 -> [w373 _]
          frame False {
            n152 = Bundle By Name(cluster=w382, "configuration.Search Paths"=w381) -> (w374:T19)
            n153 = call <vilib>:"save cache.vi"("error in"=w375, "cache"=w374, "path"=w373) -> ("error out"=w376:errorcluster)  [unwired: 8 in]
            n154 = call <vilib>:"Send Local Message.vi"("message queue in"=w378, "message name"="FindPluginNodes", "message value"="Refresh", "error in"=w376) -> ("error out"=w377:errorcluster)  [unwired: 9 in, 2 out]
          }
          frame True {
          }
        }
      }
      frame "FindPluginNodes" {
        n155 = Unbundle By Name(w401) -> ("SplashScreen"=w391:T4, "classes cache"=w387:path)
        n156 = flat-sequence {
          tunnel: w398 -> [w402]
          tunnel: [w402] -> w397
          frame #0 {
            n157 = call <vilib>:"Set Busy.vi"() -> ()  [unwired: 10 in, 2 out]
          }
        }
        n158 = Equal?(x="Refresh", y=w400) -> (x = y?=w392:bool)
        n159 = call <vilib>:"load cache.vi"("error in"=w397, "cache path"=w387) -> ("error out"=w396:errorcluster, "cache"=w395:T19)  [unwired: 8 in]
        n160 = case shown="No Error" w396 {
          selector: w396 -> [w406 w407]
          tunnel: [w404 w408] -> w393
          tunnel: w395 -> [w405 _]
          tunnel: [w406 _] -> w394
          frame No Error {
            n161 = call <vilib>:"remove missing files.vi"("cache in"=w405) -> ("cache out"=w404:T19)  [unwired: 10 in]
          }
          frame Error {
            n162 = call <vilib>:"create default cache.vi"() -> ("cache"=w408:T19)  [unwired: 11 in]
            n163 = call <vilib>:"Clear Errors.vi"("error in (no error)"=w407) -> ()  [unwired: 6 in, 1 out]
          }
        }
        n164 = call <vilib>:"identify new classes.vi"("error in"=w394, "force scan"=w392, "cache in"=w393) -> ("error out"=w388:errorcluster, "cache out"=w384:T19)  [unwired: 7 in]
        n165 = call "Update.vi"("Update"=T14 {"Text"="Loading Classes...", "percent"=45.0}, "SplashScreen in"=w391) -> ("error out"=w390:errorcluster)  [unwired: 8 in, 1 out]
        n166 = call <vilib>:"Clear Errors.vi"("error in (no error)"=w390) -> ()  [unwired: 6 in, 1 out]
        n167 = call <vilib>:"save cache.vi"("error in"=w388, "cache"=w384, "path"=w387) -> ("error out"=w386:errorcluster)  [unwired: 8 in]
        n168 = flat-sequence {
          tunnel: w386 -> [w403]
          tunnel: [w403] -> w385
          frame #0 {
            n169 = call <vilib>:"Unset Busy.vi"() -> ()  [unwired: 11 in, 1 out]
          }
        }
      }
      frame "Test" {
        n170 = in-place {
          in-place-border: w415 -> [w427]
          in-place-border: [w422] -> w409
          n171 = in-place-cluster #4(w412) -> ("repository"=w417:refnum<class "SystemConfigRepo.lvclass">, "root"=w424:T3)
          n172 = call-dynamic "ReadTree.vi"("error in"=w427, "root"=w424, "repository in"=w417) -> ("error out"=w423:errorcluster, "repository out"=w419:refnum<class "NISE_CEF_Repository.lvclass">)  [unwired: 7 in]
          n173 = To More Specific Class(target class=w417, reference=w419, error in=w423) -> (specific class reference=w418:refnum<class "SystemConfigRepo.lvclass">, error out=w420:errorcluster)
          n174 = call-dynamic "WriteTree.vi"("error in"=w420, "repository in"=w418) -> ("error out"=w426:errorcluster, "root"=w425:T3, "repository out"=w421:refnum<class "NISE_CEF_Repository.lvclass">)  [unwired: 7 in]
          n175 = To More Specific Class(target class=w417, reference=w421, error in=w426) -> (specific class reference=w416:refnum<class "SystemConfigRepo.lvclass">, error out=w422:errorcluster)
          n176 = in-place-cluster #4("repository"=w416, "root"=w425) -> (w411:T2)
        }
        n177 = call <vilib>:"Send Local Message.vi"("message queue in"=w413, "message name"="PopulateTree", "error in"=w409) -> ("error out"=w414:errorcluster)  [unwired: 10 in, 2 out]
      }
      frame "HandleMenu" {
        n178 = Unflatten From String(type=T15 {"node id"="", "RightClickPath"=""} ("input cluster"), binary string=w451, error in (no error)=w452) -> (value=w449:T15, error out=w448:errorcluster)  [unwired: 2 in, 1 out]
        n179 = Unbundle By Name(w449) -> ("RightClickPath"=w444:string, "node id"=w447:string)
        n180 = call <vilib>:"IDtoNode.vi"("error in"=w448, "ID"=w447) -> ("error out"=w446:errorcluster, "node ref"=w433:T3)  [unwired: 7 in, 1 out]
        n181 = in-place {
          in-place-border: w446 -> [w479]
          in-place-border: [w476] -> w439
          in-place-border: [w475] -> w445
          in-place-border: w444 -> [w474]
          in-place-border: [w474] -> w443
          in-place-border: w442 -> [w473]
          in-place-border: w441 -> [w472]
          in-place-border: [w469] -> w435
          in-place-border: [w468] -> w430
          n182 = in-place-dvr #5(w433) -> (w470:refnum<class "NISE_CEF_Node.lvclass">, w478:errorcluster)
          n183 = Merge Errors(w479, w478) -> (w477:errorcluster)
          n184 = call-dynamic "MenuHandler.vi"("tree control"=w472, "main message queue"=w473, "error in"=w477, "menu string"=w474, "NISE_CEF_Node in"=w470) -> ("error out"=w476:errorcluster, "refresh tree?"=w468:bool, "Unhandled"=w475:bool, "NISE_CEF_Node out"=w471:refnum<class "NISE_CEF_Node.lvclass">)  [unwired: 3 in]
          n185 = Not Equal?(x=w470, y=w471) -> (x != y?=w469:bool)
          n186 = in-place-dvr #5(w471) -> (w428:T3, w431:errorcluster)
        }
        n187 = Unbundle By Name(w438) -> ("unsaved changes"=w436:bool, "standard events.node change"=w429:T7)
        n188 = Merge Errors(w431, w439) -> (w432:errorcluster)
        n189 = case shown="False" w445 {
          tunnel: w443 -> [_ w463]
          tunnel: [w456 w465] -> w440
          tunnel: w432 -> [w457 w464]
          tunnel: w430 -> [w455 _]
          tunnel: w429 -> [w454 _]
          tunnel: w428 -> [w453 _]
          frame False {
            n190 = case shown="False" w455 {
              tunnel: w457 -> [w458 w462]
              tunnel: [w458 w461] -> w456
              tunnel: w454 -> [_ w460]
              tunnel: w453 -> [_ w459]
              frame False {
              }
              frame True {
                n191 = Generate User Event(user event=w460, event data cluster=w459, error in=w462) -> (error out=w461:errorcluster)  [unwired: 1 in, 1 out]
              }
            }
          }
          frame True {
            n192 = call <vilib>:"NISE_error generator.vi"("error in"=w464, "source"="configuration tool main.vi", "append error message"=w463, "error code (0)"=538506) -> ("error out"=w465:errorcluster)  [unwired: 5 in]
          }
        }
        n193 = Or(x=w436, y=w435) -> (x .or. y?=w434:bool)
        n194 = Bundle By Name(cluster=w438, "unsaved changes"=w434) -> (w437:T2)
      }
      frame "Script Include VI" {
        n195 = call "call include vi script.vi"("error in (no error)"=w481, "state cluster"=w482) -> ("error out"=w480:errorcluster)  [unwired: 9 in]
      }
      frame "-------TreeControl Operations-----------" {
        # "Dummy case to add a seperation in the Case Structure menu"
      }
      frame "AddNode" {
        n196 = call <vilib>:"Set Busy.vi"() -> ("error out"=w492:errorcluster)  [unwired: 10 in, 1 out]
        n197 = flat-sequence {
          tunnel: w511 -> [w513]
          tunnel: [w513] -> w498
          tunnel: w492 -> [_]
          frame #0 {
          }
        }
        n198 = Unflatten From String(type=T16 {"node type"="", "to add to"=""} ("input cluster"), binary string=w512) -> (value=w506:T16)  [unwired: 3 in, 2 out]
        n199 = Unbundle By Name(w506) -> ("to add to"=w504:string, "node type"=w501:string)
        n200 = in-place {
          in-place-border: w501 -> [w519]
          in-place-border: [w516] -> w500
          in-place-border: w498 -> [w515]
          in-place-border: [w514] -> w499
          n201 = in-place-cluster #6(w510) -> ("repository"=w518:refnum<class "SystemConfigRepo.lvclass">)
          n202 = call-dynamic "GetClassPath.vi"("error in"=w515, "class name"=w519, "Repository in"=w518) -> ("error out"=w514:errorcluster, "class path"=w516:path, "Repository out"=w517:refnum<class "SystemConfigRepo.lvclass">)  [unwired: 6 in]
          n203 = in-place-cluster #6("repository"=w517) -> (w494:T2)
        }
        n204 = Unbundle By Name(w494) -> ("glyph manager"=w486:T11)
        n205 = call <vilib>:"Get LV Class Default Value.vi"("error in (no error)"=w499, "class path"=w500) -> ("error out"=w508:errorcluster, "object"=w509:refnum<class>)  [unwired: 8 in]
        n206 = To More Specific Class(target class=refnum<class "NISE_CEF_Node.lvclass"> refnum ("NISE_CEF_Node.lvclass"), reference=w509, error in=w508) -> (specific class reference=w489:refnum<class "NISE_CEF_Node.lvclass">, error out=w490:errorcluster)
        n207 = call-dynamic "AddGlyphtoGManager.vi"("error in"=w490, "glyph manager"=w486, "NISE_CEF_Node in"=w489) -> ("error out"=w487:errorcluster, "glyph manager out"=w485:T11, "NISE_CEF_Node out"=w488:refnum<class "NISE_CEF_Node.lvclass">)  [unwired: 6 in]
        n208 = call <vilib>:"AddNode.vi"("error in"=w487, "node in"=w488, "parent node ID"=w504) -> ("error out"=w503:errorcluster, "summary"=w502:T25[])  [unwired: 7 in]
        n209 = call <vilib>:"PopulateTreeSumaryWithGlyphManager.vi"("error in"=w503, "glyph manager"=w485, "summary"=w502, "tree ref in"=w497) -> ("error out"=w493:errorcluster, "glyph manager out"=w491:T11)  [unwired: 6 in]
        n210 = Bundle By Name(cluster=w494, "unsaved changes"=TRUE, "glyph manager"=w491) -> (w496:T2)
        n211 = flat-sequence {
          tunnel: w493 -> [_]
          frame #0 {
            n212 = call <vilib>:"Unset Busy.vi"() -> ()  [unwired: 11 in, 1 out]
          }
        }
      }
      frame "Duplicate" {
        n213 = Unbundle By Name(w522) -> ("glyph manager"=w521:T11)
        n214 = call <vilib>:"IDtoNode.vi"("error in"=w529, "ID"=w530) -> ("error out"=w527:errorcluster, "invalid Id"=w526:bool, "node ref"=w528:T3)  [unwired: 7 in]
        n215 = case shown="False" w526 {
          tunnel: [w543 w545] -> w531
          tunnel: w528 -> [w542 _]
          tunnel: w527 -> [w539 w545]
          tunnel: w525 -> [w535 _]
          tunnel: w521 -> [w533 w544]
          tunnel: [w534 w544] -> w520
          frame False {
            n216 = call <vilib>:"DuplicateNode.vi"("same parent?"=TRUE ("s"), "error in"=w539, "node ref in"=w542) -> ("error out"=w540:errorcluster, "new node ref"=w541:T3)  [unwired: 7 in]
            n217 = call <vilib>:"SummaryWithGlyphManager.vi"("error in"=w540, "glyph manager"=w533, "node self ref"=w541) -> ("error out"=w537:errorcluster, "glyph manager out"=w532:T11, "summary"=w536:T25[])  [unwired: 6 in]
            n218 = call <vilib>:"PopulateTreeSumaryWithGlyphManager.vi"("error in"=w537, "glyph manager"=w532, "summary"=w536, "tree ref in"=w535) -> ("error out"=w543:errorcluster, "glyph manager out"=w534:T11)  [unwired: 6 in]
          }
          frame True {
          }
        }
        n219 = Bundle By Name(cluster=w522, "unsaved changes"=TRUE, "glyph manager"=w520) -> (w524:T2)
      }
      frame "RefreshNode" {
        # "Refreshes the node in the Tree               Sets the save flag to true                       This case can be called from the UIs of the nodes"
        n220 = Unbundle By Name(w548) -> ("glyph manager"=w547:T11)
        n221 = call <vilib>:"IDtoNode.vi"("error in"=w554, "ID"=w553) -> ("error out"=w552:errorcluster, "invalid Id"=w550:bool, "node ref"=w551:T3)  [unwired: 7 in]
        n222 = case shown="False" w550 {
          tunnel: [w565 w567] -> w556
          tunnel: w552 -> [w562 w567]
          tunnel: w551 -> [w561 _]
          tunnel: w549 -> [w560 _]
          tunnel: w547 -> [w558 w566]
          tunnel: [w559 w566] -> w546
          frame False {
            n223 = call <vilib>:"SummaryWithGlyphManager.vi"("error in"=w562, "glyph manager"=w558, "node self ref"=w561) -> ("error out"=w564:errorcluster, "glyph manager out"=w557:T11, "summary"=w563:T25[])  [unwired: 6 in]
            n224 = call <vilib>:"RefreshSubTreeWithGlyphManager.vi"("error in"=w564, "glyph manager"=w557, "node information"=w563, "tree ref in"=w560) -> ("error out"=w565:errorcluster, "glyph manager out"=w559:T11)  [unwired: 5 in, 1 out]
          }
          frame True {
          }
        }
        n225 = Bundle By Name(cluster=w548, "glyph manager"=w546) -> (w555:T2)
      }
      frame "SetDirtyDot" {
        n226 = Bundle By Name(cluster=w571, "unsaved changes"=TRUE ("SaveFlag")) -> (w570:T2)
      }
      frame "RemoveNode" {
        n227 = Unbundle By Name(w575) -> ("standard events"=w574:T5)
        n228 = call <vilib>:"IDtoNode.vi"("error in"=w582, "ID"=w583) -> ("error out"=w580:errorcluster, "invalid Id"=w578:bool, "node ref"=w579:T3)  [unwired: 7 in]
        n229 = case shown="False" w578 {
          tunnel: w580 -> [w591 w601]
          tunnel: w579 -> [w589 _]
          tunnel: [w593 w601] -> w581
          tunnel: w577 -> [w592 _]
          tunnel: w576 -> [w588 _]
          tunnel: w574 -> [w587 _]
          frame False {
            n230 = call "check if subpanel should be closed.vi"("error in"=w591, "SubPanel in"=w588, "node in"=w589) -> ("error out"=w586:errorcluster, "needs closing"=w584:bool, "node out"=w590:T3)  [unwired: 6 in]
            n231 = case shown="True" w584 {
              tunnel: w588 -> [_ w600]
              tunnel: w587 -> [_ w597]
              tunnel: w586 -> [w596 w599]
              tunnel: [w596 w598] -> w585
              frame False {
              }
              frame True {
                n232 = call "Remove UI without races.vi"("error in"=w599, "standard events"=w597, "sub panel ref in"=w600) -> ("error out"=w598:errorcluster)  [unwired: 7 in, 1 out]
              }
            }
            n233 = call <vilib>:"RemoveNode.vi"("error in"=w585, "node"=w590) -> ("error out"=w594:errorcluster, "node ID"=w595:string)  [unwired: 8 in]
            n234 = call <vilib>:"ClearTreeNode.vi"("error in"=w594, "tag"=w595, "tree reference"=w592) -> ("error out"=w593:errorcluster)  [unwired: 8 in]
          }
          frame True {
          }
        }
        n235 = Bundle By Name(cluster=w575, "unsaved changes"=TRUE) -> (w573:T2)
      }
      frame "PopulateTree" {
        n236 = Unbundle By Name(w621) -> ("current path"=w610:path, "glyph manager"=w603:T11, "root"=w618:T3)
        n237 = call <vilib>:"SummaryWithGlyphManager.vi"("error in"=w616, "glyph manager"=w603, "depth"=0 ("Depth"), "node self ref"=w618) -> ("error out"=w619:errorcluster, "glyph manager out"=w602:T11, "summary"=w620:T25[])  [unwired: 5 in]
        n238 = call <vilib>:"Check if File or Folder Exists.vi"("path"=w610) -> ("file or folder exists?"=w606:bool, "dup path"=w609:path)  [unwired: 8 in, 1 out]
        n239 = call <vilib>:"RefreshEntireTreeWithGlyphManager.vi"("calling VI in"=w612, "error in"=w619, "glyph manager"=w602, "array"=w620, "tree ref in"=w615) -> ("error out"=w614:errorcluster, "glyph manager out"=w604:T11)  [unwired: 5 in]
        n240 = Strip Path(path=w609) -> (name=w608:string)  [unwired: 1 out]
        n241 = Select(t=w608, s=w606, f="Tag Bus Configuration editor") -> (s? t:f=w607:string)
        n242 = Bundle By Name(cluster=w621, "glyph manager"=w604) -> (w605:T2)
        n243 = property class="VI"(reference=w612, error in=w614, "Front Panel.Title"=w607) -> (error out=w613:errorcluster)  [unwired: 1 out]
      }
      frame "CleansubPanel" {
        n244 = Unbundle By Name(w625) -> ("standard events"=w622:T5)
        n245 = call "Remove UI without races.vi"("error in"=w626, "standard events"=w622, "sub panel ref in"=w623) -> ("error out"=w624:errorcluster)  [unwired: 7 in, 1 out]
      }
      frame "ActivateNode" {
        n246 = Unbundle By Name(w634) -> ("standard events"=w631:T5)
        n247 = call <vilib>:"Set Busy.vi"("error in (no error)"=w637) -> ("error out"=w629:errorcluster)  [unwired: 9 in, 1 out]
        n248 = call <vilib>:"IDtoNode.vi"("error in"=w629, "ID"=w638) -> ("error out"=w630:errorcluster, "invalid Id"=w633:bool, "node ref"=w632:T3)  [unwired: 7 in]
        n249 = case shown="False" w633 {
          tunnel: w632 -> [w645 _]
          tunnel: [w646 w649] -> w628
          tunnel: w630 -> [w643 w650]
          tunnel: w635 -> [w642 _]
          tunnel: w631 -> [w639 w647]
          tunnel: w627 -> [w640 w648]
          frame False {
            n250 = call "Remove UI without races.vi"("error in"=w643, "standard events"=w639, "sub panel ref in"=w640) -> ("error out"=w644:errorcluster, "sub panel ref out"=w641:refnum<vi>)  [unwired: 7 in]
            n251 = call <vilib>:"LoadNodeUIStandardEvents.vi"("user event out"=w639, "error in"=w644, "sub panel ref in"=w641, "main queue"=w642, "node"=w645) -> ("error out"=w646:errorcluster)  [unwired: 6 in]
          }
          frame True {
            n252 = call "Remove UI without races.vi"("error in"=w650, "standard events"=w647, "sub panel ref in"=w648) -> ("error out"=w649:errorcluster)  [unwired: 7 in, 1 out]
          }
        }
        n253 = call <vilib>:"Unset Busy.vi"("error in (no error)"=w628) -> ("error out"=w636:errorcluster)  [unwired: 10 in]
      }
      frame "Move" {
        n254 = Unflatten From String(type=T17 {"node ref"=refnum, "new parent"=refnum} ("Cluster"), binary string=w663, error in (no error)=w662) -> (value=w658:T17, error out=w657:errorcluster)  [unwired: 2 in, 1 out]
        n255 = Unbundle By Name(w658) -> ("node ref"=w654:T3, "new parent"=w653:T3)
        n256 = call <vilib>:"MoveNode.vi"("error in"=w657, "new parent"=w653, "node"=w654) -> ("error out"=w655:errorcluster)  [unwired: 8 in]
        n257 = call <vilib>:"Send Local Message.vi"("message queue in"=w660, "message name"="PopulateTree", "error in"=w655) -> ("error out"=w661:errorcluster)  [unwired: 10 in, 2 out]
        n258 = Bundle By Name(cluster=w664, "unsaved changes"=TRUE) -> (w652:T2)
      }
      frame "RefreshNodeView" {
        # "This user event is used by editor nodes to update their subpanels when data in the tree changes."
        n259 = Unbundle By Name(w668) -> ("standard events.refresh UI"=w666:T9)
        n260 = Generate User Event(user event=w666, event data cluster=TRUE ("event data"), error in=w669) -> (error out=w667:errorcluster)  [unwired: 1 in, 1 out]
      }
      frame "NodeDataChange" {
        n261 = call <vilib>:"Send Local Message.vi"("message queue in"=w673, "message name"="RefreshNode", "message value"=w672, "error in"=w675) -> ("error out"=w674:errorcluster)  [unwired: 9 in, 2 out]
        n262 = Bundle By Name(cluster=w677, "unsaved changes"=TRUE) -> (w671:T2)
      }
    }
  }
  n263 = while "User Interface Event Handler" {
    tunnel: w20 -> [w684]
    tunnel: w7 -> [w680]
    tunnel: w5 -> [w679]
    tunnel: [w678] -> w3
    stop <- w683 stop-if-true
    n264 = event shown="[2] \"View\": Shortcut Menu Selection (User)" {
      selector: w679 -> [_ _ _ _ _ _ _ _ _ _]
      dyn-events: [_ _ _ _ _ _ _ _ _ _] -> w678
      timeout: _ -> [_ _ _ _ _ _ _ _ _ _]
      tunnel: w684 -> [w692 w711 w723 w765 w805 w812 w839 w843 w853 w858]
      tunnel: [_ _ _ _ TRUE _ _ _ _ _] -> w683
      tunnel: [w692 w710 w715 w767 w801 w812 w836 w843 w851 w857] -> w682
      tunnel: [w687 _ w716 w766 w802 w808 w835 w840 w849 w855] -> w681
      tunnel: w680 -> [w691 _ w721 w764 w803 w811 w834 w842 w850 w856]
      event "View": Shortcut Menu Activation? {
        n265 = event-data() -> ("CtlRef"=w698:refnum<vi>, "Coords"=w697:T26, "MenuRef"=w694:refnum<k9>)  [unwired: 1 in]
        n266 = invoke class="Tree (strict)" method="Point To Row Column"(reference=w698, error in=w691, "Point"=w697) -> (error out=w690:errorcluster, "Tag"=w696:string)  [unwired: 5 in, 6 out]
        n267 = call <vilib>:"IDtoNode.vi"("error in"=w690, "ID"=w696) -> ("error out"=w688:errorcluster, "invalid Id"=w693:bool, "node ref"=w695:T3)  [unwired: 7 in]
        n268 = case shown="False" w693 {
          selector: w693 -> [_ w708]
          tunnel: w695 -> [w702 _]
          tunnel: w694 -> [w701 _]
          tunnel: [w700 _] -> w689
          tunnel: [w699 _] -> w686
          tunnel: [_ w708] -> w685
          frame False {
            n269 = in-place {
              in-place-border: w701 -> [w705]
              in-place-border: [w703] -> w700
              n270 = in-place-dvr #7(w702) -> (w707:refnum<class "NISE_CEF_Node.lvclass">, w704:errorcluster)
              n271 = call-dynamic "ShortcutMenu.vi"("error in"=w704, "menu ref in"=w705, "node in"=w707) -> ("error out"=w703:errorcluster, "node out"=w706:refnum<class "NISE_CEF_Node.lvclass">)  [unwired: 6 in, 1 out]
              n272 = in-place-dvr #7(w706) -> (w699:errorcluster)  [unwired: 1 out]
            }
          }
          frame True {
          }
        }
        n273 = Merge Errors(w686, w689, w688) -> (w687:errorcluster)
        n274 = event-data("Discard?"=w685) -> ()  [unwired: 1 in, 1 out]
      }
      event User Event {
        n275 = event-data() -> ("node ref"=w713:T3)  [unwired: 1 in]
        n276 = call <vilib>:"NodetoID.vi"("node ref"=w713) -> ("ID"=w709:string)  [unwired: 9 in, 1 out]
        n277 = call <vilib>:"Send Local Message.vi"("message queue in"=w711, "message name"="NodeDataChange", "message value"=w709) -> ("message queue out"=w710:T13)  [unwired: 10 in, 2 out]
      }
      event "View": Shortcut Menu Selection (User) {
        # "=nodeID"
        n278 = event-data() -> ("ItemPath"=w719:string, "CtlRef"=w726:refnum<vi>, "Coords"=w727:T26)  [unwired: 1 in]
        n279 = invoke class="Tree (strict)" method="Point To Row Column"(reference=w726, error in=w721, "Point"=w727) -> (error out=w720:errorcluster, "Tag"=w722:string)  [unwired: 5 in, 6 out]
        n280 = Match Pattern(string=w719, regular expression=":") -> (before substring=w725:string, after substring=w724:string)  [unwired: 1 in, 2 out]
        n281 = case shown="Default" w725 {
          tunnel: w724 -> [_ _ _ w756]
          tunnel: w723 -> [w734 w745 w751 w758]
          tunnel: w722 -> [w732 w739 w749 w757]
          tunnel: [w731 w743 w748 w754] -> w718
          tunnel: [w730 w742 w746 w752] -> w717
          tunnel: w720 -> [w729 w738 w747 w753]
          tunnel: w719 -> [_ w735 _ _]
          frame "Remove" {
            n282 = call <vilib>:"Send Local Message.vi"("message queue in"=w734, "message name"="RemoveNode" ("Message Name"), "message value"=w732, "error in"=w729) -> ("message queue out"=w731:T13, "error out"=w730:errorcluster)  [unwired: 9 in, 1 out]
          }
          frame Default {
            n283 = Bundle By Name(cluster=T15 {"node id"="", "RightClickPath"=""} ("input cluster"), "node id"=w739, "RightClickPath"=w735) -> (w740:T15)
            n284 = Flatten To String(anything=w740, error in (no error)=w738) -> (data string=w736:string, error out=w737:errorcluster)  [unwired: 2 in, 1 out]
            n285 = call <vilib>:"Send Local Message.vi"("message queue in"=w745, "message name"="HandleMenu" ("Message Name"), "message value"=w736, "error in"=w737) -> ("message queue out"=w743:T13, "error out"=w742:errorcluster)  [unwired: 9 in, 1 out]
          }
          frame "Duplicate" {
            n286 = call <vilib>:"Send Local Message.vi"("message queue in"=w751, "message name"="Duplicate" ("Message Name"), "message value"=w749, "error in"=w747) -> ("message queue out"=w748:T13, "error out"=w746:errorcluster)  [unwired: 9 in, 1 out]
          }
          frame "Add" {
            n287 = Bundle By Name(cluster=T16 {"node type"="", "to add to"=""} ("input cluster"), "node type"=w756, "to add to"=w757) -> (w759:T16)
            n288 = Flatten To String(anything=w759) -> (data string=w760:string)  [unwired: 3 in, 2 out]
            n289 = call <vilib>:"Send Local Message.vi"("message queue in"=w758, "message name"="AddNode" ("Message Name"), "message value"=w760, "error in"=w753) -> ("message queue out"=w754:T13, "error out"=w752:errorcluster)  [unwired: 9 in, 1 out]
          }
        }
        n290 = call <vilib>:"Send Local Message.vi"("message queue in"=w718, "message name"="RefreshNodeView", "error in"=w717) -> ("message queue out"=w715:T13, "error out"=w716:errorcluster)  [unwired: 10 in, 1 out]
      }
      event "View": Drop {
        n291 = event-data() -> ("CtlRef"=w763:refnum<vi>, "Coords"=w762:T26)  [unwired: 1 in]
        n292 = invoke class="Tree (strict)" method="Point To Row Column"(reference=w763, error in=w764, "Point"=w762) -> (reference out=w781:refnum<vi>, error out=w780:errorcluster, "Tag"=w777:string)  [unwired: 5 in, 5 out]
        n293 = call <vilib>:"ValidDragDrop.vi"("error in"=w780, "drag over"=w777, "tree ref in"=w781) -> ("error out"=w772:errorcluster, "accepted"=w775:bool, "drag"=w779:string, "tree ref out"=w782:refnum<vi>)  [unwired: 5 in]
        n294 = call <vilib>:"IDtoNode.vi"("error in"=w772, "ID"=w777) -> ("error out"=w773:errorcluster, "invalid Id"=w770:bool, "node ref"=w776:T3)  [unwired: 7 in]
        n295 = call <vilib>:"IDtoNode.vi"("error in"=w773, "ID"=w779) -> ("error out"=w771:errorcluster, "invalid Id"=w769:bool, "node ref"=w778:T3)  [unwired: 7 in]
        n296 = Compound Arithmetic op=AND(w775, invert w770, invert w769) -> (w774:bool)
        n297 = case shown="True" w774 {
          tunnel: w779 -> [_ w798]
          tunnel: w782 -> [_ w800]
          tunnel: [_ TRUE] -> w768
          tunnel: w777 -> [_ w796]
          tunnel: w765 -> [w784 w785]
          tunnel: [w784 w792] -> w767
          tunnel: [w783 w791] -> w766
          tunnel: w778 -> [_ w787]
          tunnel: w776 -> [_ w786]
          tunnel: w771 -> [w783 w788]
          frame False {
          }
          frame True {
            n298 = invoke class="Tree (strict)" method="Edit Tree Items.Move Item"(reference=w800, error in=w788, "tag"=w798, "New Parent"=w796) -> (error out=w789:errorcluster)  [unwired: 3 in, 6 out]
            n299 = Bundle By Name(cluster=T17 {"node ref"=refnum, "new parent"=refnum} ("Cluster"), "new parent"=w786, "node ref"=w787) -> (w795:T17)
            n300 = Flatten To String(anything=w795, error in (no error)=w789) -> (data string=w794:string, error out=w790:errorcluster)  [unwired: 2 in, 1 out]
            n301 = call <vilib>:"Send Local Message.vi"("message queue in"=w785, "message name"="Move", "message value"=w794, "error in"=w790) -> ("message queue out"=w792:T13, "error out"=w791:errorcluster)  [unwired: 9 in, 1 out]
          }
        }
        n302 = event-data("Accepted?"=w768) -> ()  [unwired: 1 in, 1 out]
      }
      event "Exit": Value Change {
        # "Exit the application                                           >> Stop this message generator loop    Cleaning errors if the other loop stop this one"
        n303 = event-data() -> ()  [unwired: 1 in, 1 out]
        n304 = call <vilib>:"Send Local Message.vi"("message queue in"=w805, "message name"="Close", "error in"=w803) -> ("message queue out"=w801:T13, "error out"=w806:errorcluster)  [unwired: 10 in, 1 out]
        n305 = call <vilib>:"Clear Errors.vi"("error in (no error)"=w806) -> ("error out"=w802:errorcluster)  [unwired: 6 in]
      }
      event "View": Drag Starting? {
        n306 = event-data() -> ("Data"=w818:T27, "CtlRef"=w820:refnum<vi>, "Coords"=w819:T26)  [unwired: 1 in]
        n307 = invoke class="Tree (strict)" method="Point To Row Column"(reference=w820, error in=w811, "Point"=w819) -> (error out=w810:errorcluster, "Tag"=w817:string)  [unwired: 5 in, 6 out]
        n308 = call <vilib>:"IDtoNode.vi"("error in"=w810, "ID"=w817) -> ("error out"=w809:errorcluster, "invalid Id"=w816:bool, "node ref"=w815:T3)  [unwired: 7 in]
        n309 = case shown="False" w816 {
          tunnel: w815 -> [w826 _]
          tunnel: [w823 TRUE ("Removable")] -> w813
          tunnel: w809 -> [w822 w832]
          tunnel: [w821 w832] -> w808
          frame False {
            n310 = in-place {
              in-place-border: [w829] -> w825
              in-place-border: w822 -> [w828]
              in-place-border: [w827] -> w821
              n311 = in-place-dvr #8(w826) -> (w831:refnum<class "NISE_CEF_Node.lvclass">)  [unwired: 1 out]
              n312 = call-dynamic "EditOptions.vi"("error in"=w828, "node in"=w831) -> ("error out"=w827:errorcluster, "edit options"=w829:T28, "node out"=w830:refnum<class "NISE_CEF_Node.lvclass">)  [unwired: 6 in, 1 out]
              n313 = in-place-dvr #8(w830) -> ()  [unwired: 2 out]
            }
            n314 = Unbundle By Name(w825) -> ("movable"=w824:bool)
            n315 = Not(x=w824) -> (.not. x?=w823:bool)
          }
          frame True {
          }
        }
        n316 = event-data("Data"=w818, "Drag Mode"=enum32{"copy or move", "copy only", "move only"}."move only", "Discard?"=w813) -> ()  [unwired: 1 in, 1 out]
      }
      event "View": Value Change {
        n317 = event-data() -> ("NewVal"=w837:string)  [unwired: 1 in]
        n318 = call <vilib>:"Send Local Message.vi"("message queue in"=w839, "message name"="ActivateNode" ("Message Name"), "message value"=w837, "error in"=w834) -> ("message queue out"=w836:T13, "error out"=w835:errorcluster)  [unwired: 9 in, 1 out]
      }
      event "View": event type 3.0.xa000003a {
        n319 = event-data() -> ("CtlRef"=w848:refnum<vi>, "Coords"=w845:T26)  [unwired: 1 in]
        n320 = invoke class="Tree (strict)" method="Point To Row Column"(reference=w848, error in=w842, "Point"=w845) -> (reference out=w847:refnum<vi>, error out=w841:errorcluster, "Tag"=w846:string)  [unwired: 5 in, 5 out]
        n321 = call <vilib>:"ValidDragDrop.vi"("error in"=w841, "drag over"=w846, "tree ref in"=w847) -> ("error out"=w840:errorcluster, "accepted"=w844:bool)  [unwired: 5 in, 2 out]
        n322 = event-data("Accepted?"=w844) -> ()  [unwired: 1 in, 1 out]
      }
      event Panel Close? {
        # "Intercepts the upper right close panel operation to allow a smooth shutdown as opposed to immediately killing the app."
        n323 = event-data() -> ()  [unwired: 1 in, 1 out]
        n324 = call <vilib>:"Send Local Message.vi"("message queue in"=w853, "message name"="Close?", "error in"=w850) -> ("message queue out"=w851:T13, "error out"=w849:errorcluster)  [unwired: 10 in, 1 out]
        n325 = event-data("Discard?"=TRUE) -> ()  [unwired: 1 in, 1 out]
      }
      event Menu Selection (User) {
        n326 = event-data() -> ("ItemPath"=w859:string)  [unwired: 1 in]
        n327 = case shown="\"_Tools:Script Include VI\"" w859 {
          tunnel: w858 -> [w861 w867 w872 w877 w882 w887 w896 w901 w906 w911 w916 w921 w927 w931]
          tunnel: [w861 w863 w868 w873 w878 w883 w893 w898 w903 w908 w913 w918 w924 w930] -> w857
          tunnel: w856 -> [w860 w865 w870 w875 w880 w885 w892 w899 w904 w909 w914 w919 w925 w929]
          tunnel: [w860 w864 w869 w874 w879 w884 w890 w897 w902 w907 w912 w917 w923 w928] -> w855
          frame Default {
            n328 = One Button Dialog(message="Unknown Menu Option") -> ()  [unwired: 1 in, 1 out]
          }
          frame "_File:_New" {
            n329 = call <vilib>:"Send Local Message.vi"("message queue in"=w867, "message name"="New?" ("Message Name"), "error in"=w865) -> ("message queue out"=w863:T13, "error out"=w864:errorcluster)  [unwired: 10 in, 1 out]
          }
          frame "_File:_Open" {
            n330 = call <vilib>:"Send Local Message.vi"("message queue in"=w872, "message name"="Open?" ("Message Name"), "error in"=w870) -> ("message queue out"=w868:T13, "error out"=w869:errorcluster)  [unwired: 10 in, 1 out]
          }
          frame "_File:_Save" {
            n331 = call <vilib>:"Send Local Message.vi"("message queue in"=w877, "message name"="Save" ("Message Name"), "error in"=w875) -> ("message queue out"=w873:T13, "error out"=w874:errorcluster)  [unwired: 10 in, 1 out]
          }
          frame "_File:Save As..." {
            n332 = call <vilib>:"Send Local Message.vi"("message queue in"=w882, "message name"="SaveAs" ("Message Name"), "error in"=w880) -> ("message queue out"=w878:T13, "error out"=w879:errorcluster)  [unwired: 10 in, 1 out]
          }
          frame "_File:_Exit" {
            n333 = call <vilib>:"Send Local Message.vi"("message queue in"=w887, "message name"="Close?" ("Message Name"), "error in"=w885) -> ("message queue out"=w883:T13, "error out"=w884:errorcluster)  [unwired: 10 in, 1 out]
          }
          frame "_Tools:Multiple Parameter Editor" {
            n334 = call <vilib>:"Send Local Message.vi"("message queue in"=w896, "message name"="CleansubPanel", "error in"=w892) -> ("message queue out"=w895:T13, "error out"=w891:errorcluster)  [unwired: 10 in, 1 out]
            n335 = call <vilib>:"Send Local Message.vi"("message queue in"=w895, "message name"="Custom View", "message value"="Multiple Parameter Editor" ("Message Name"), "error in"=w891) -> ("message queue out"=w893:T13, "error out"=w890:errorcluster)  [unwired: 9 in, 1 out]
          }
          frame "_Tools:Test" {
            n336 = call <vilib>:"Send Local Message.vi"("message queue in"=w901, "message name"="Test", "error in"=w899) -> ("message queue out"=w898:T13, "error out"=w897:errorcluster)  [unwired: 10 in, 1 out]
          }
          frame "_Tools:Deploy Tool" {
            n337 = call <vilib>:"Send Local Message.vi"("message queue in"=w906, "message name"="DeployTool", "error in"=w904) -> ("message queue out"=w903:T13, "error out"=w902:errorcluster)  [unwired: 10 in, 1 out]
          }
          frame "_Tools:Save Binary" {
            n338 = call <vilib>:"Send Local Message.vi"("message queue in"=w911, "message name"="Save Binary", "error in"=w909) -> ("message queue out"=w908:T13, "error out"=w907:errorcluster)  [unwired: 10 in, 1 out]
          }
          frame "_Tools:Script Include VI" {
            n339 = call <vilib>:"Send Local Message.vi"("message queue in"=w916, "message name"="Script Include VI", "error in"=w914) -> ("message queue out"=w913:T13, "error out"=w912:errorcluster)  [unwired: 10 in, 1 out]
          }
          frame "_Tools:Load Binary" {
            n340 = call <vilib>:"Send Local Message.vi"("message queue in"=w921, "message name"="Load Binary", "error in"=w919) -> ("message queue out"=w918:T13, "error out"=w917:errorcluster)  [unwired: 10 in, 1 out]
          }
          frame "_Tools:Refresh Plugins" {
            n341 = call <vilib>:"Send Local Message.vi"("message queue in"=w927, "message name"="FindPluginNodes", "message value"="Refresh", "error in"=w925) -> ("message queue out"=w924:T13, "error out"=w923:errorcluster)  [unwired: 9 in, 1 out]
          }
          frame "_Tools:Edit Plugin Search Paths" {
            n342 = call <vilib>:"Send Local Message.vi"("message queue in"=w931, "message name"="Edit Plugin Search Paths", "error in"=w929) -> ("message queue out"=w930:T13, "error out"=w928:errorcluster)  [unwired: 10 in, 1 out]
          }
        }
      }
    }
    n343 = call "send error message.vi"("error in"=w681, "message queue in"=w682) -> ()  [unwired: 9 in, 1 out]
  }
  n344 = Unregister For Events(event registration refnum=w3) -> ()  [unwired: 1 in, 1 out]
  n345 = call <vilib>:"DestroyStandardEvents.vi"("error in"=w2, "standard events"=w1) -> ()  [unwired: 9 in, 1 out]
